vi "(SubVI) Get VelocityPI.vi"(4 "axis":u32) -> (1 "Velocity (um/s)":dbl, 2 "Velocity Array":dbl[](array[numeric]) format="%.6f")   [LabVIEW 2014]
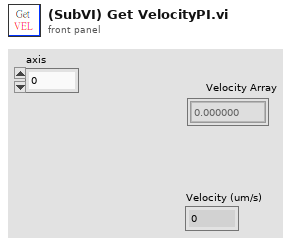
[diagram p1: front panel]
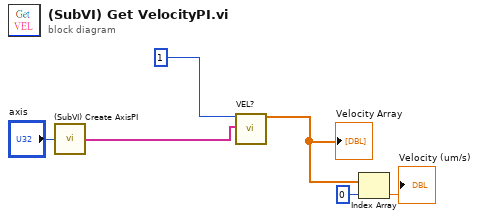
[diagram p0: block diagram]
diagram:
  n1 = call "(SubVI) Create AxisPI.vi"("axis"="axis") -> ("Axis String Array"=w5:string[])  [unwired: 2 in, 2 out]
  n2 = call "VEL?.vi"("System no."=1, "Axes to query"=w5) -> ("Velocity"=w4:dbl[])  [unwired: 3 in, 14 out]
  "Velocity Array" <- w4
  n3 = Index Array(array=w4, index=0) -> (element=→"Velocity (um/s)":dbl)
